vi "Remove Connection.vi"(8 "error in (no error)":errorcluster, 11 "Terminal in":refnum<class "Terminal.lvclass">) -> (0 "error out":errorcluster, 2 "Connection":refnum<class "Connection.lvclass">, 3 "Terminal out":refnum<class "Terminal.lvclass">)   [LabVIEW 2020, in "Terminal.lvlib" / "Terminal.lvclass"]
uses:
  Terminal.lvclass
  Terminal.lvclass/Terminal.ctl
  Connection State Callback.vi
  Data Sniffer Callback.vi
  <vilib>/IlluminatedG/lv-stream/Endpoint/Endpoint.lvclass
  <vilib>/IlluminatedG/lv-stream/Connection/Connection.lvclass
  C:/Program Files (x86)/National Instruments/LabVIEW 2020/vi.lib/IlluminatedG/lv-stream/Endpoint/Endpoint.lvclass
  C:/Program Files (x86)/National Instruments/LabVIEW 2020/vi.lib/IlluminatedG/lv-stream/Connection/Connection.lvclass
  C:/Program Files (x86)/National Instruments/LabVIEW 2020/vi.lib/IlluminatedG/IG OOPanel/OOPanel/Panel/Panel.lvclass
  C:/dev/illuminated-g/lv-stream-terminal/Terminal/Terminal/Terminal.lvclass
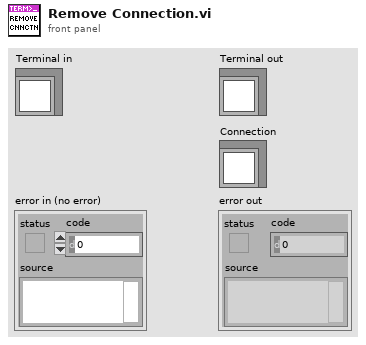
[diagram p1: front panel]
types:
  T1 = typedef "Terminal.lvlib/Terminal.lvclass/Ref Data.ctl" = cluster{"Connection":refnum<class "Connection.lvclass">, "Read Loop Running":bool, "Parse State":T2, "Terminal Options":T8, "Font Metrics":T11, "Scroll":i32, "Close Read Loop":bool, "Buffer":T7, "Pause Read Loop":bool, "User Input Enabled":bool, "Cursor Enabled":bool, "Cursor Blink":bool}
  T2 = typedef "Terminal.lvlib/Terminal.lvclass/Parse State.ctl" = cluster{"Buffer State":T3, "Cursor":T4, "Attributes":T6, "Active Buffer":T7}
  T3 = typedef "Terminal.lvlib/Terminal.lvclass/Buffer State.ctl" = cluster{"Sequence":string, "ESC":bool, "Alt Buf":bool}
  T4 = typedef "Terminal.lvlib/Terminal.lvclass/Cursor.ctl" = cluster{"Cur":T5, "Saved":T5}
  T5 = typedef "Terminal.lvlib/Terminal.lvclass/Position.ctl" = cluster{"Row":i32, "Col":i32}
  T6 = typedef "Terminal.lvlib/Text Attributes.ctl" = cluster{"FG":u32, "BG":u32, "Bold":bool, "Italic":bool, "Underline":bool, "Strike":bool, "Inverse":bool}
  T7 = typedef "Terminal.lvlib/Buffer.ctl" = enum16{"Primary", "Alternate"}
  T8 = typedef "Terminal.lvlib/Terminal Options.ctl" = cluster{"Implied CR with LF":bool, "Local Echo":bool, "Tab Width":i32, "Color Scheme":T9, "Default FG":T10, "Default BG":T10, "History Length":i32, "Font Face":string, "Font Size":i16, "Rows":i32, "Cols":i32}
  T9 = typedef "Terminal.lvlib/Color Scheme.ctl" = cluster{"Black":u32, "Red":u32, "Green":u32, "Yellow":u32, "Blue":u32, "Magenta":u32, "Cyan":u32, "White":u32, "Bright Black":u32, "Bright Red":u32, "Bright Green":u32, "Bright Yellow":u32, "Bright Blue":u32, "Bright Magenta":u32, "Bright Cyan":u32, "Bright White":u32}
  T10 = typedef "Terminal.lvlib/Color.ctl" = i8
  T11 = typedef "Terminal.lvlib/Terminal.lvclass/Font Metrics.ctl" = cluster{"Width":i16, "Height":i16}
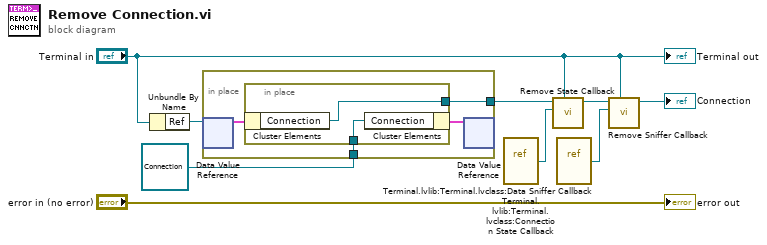
[diagram p0: block diagram]
diagram:
  n1 = Unbundle By Name("Terminal in") -> ("Ref"=w9:refnum<data-value>)
  n2 = in-place {
    in-place-border: [w11] -> w8
    in-place-border: refnum<class "Connection.lvclass"> refnum ("Connection") -> [w10]
    n3 = in-place-dvr #1(w9) -> (w13:T1)  [unwired: 1 out]
    n4 = in-place {
      in-place-border: [w15] -> w11
      in-place-border: w10 -> [w14]
      n5 = in-place-cluster #2(w13) -> ("Connection"=w15:refnum<class "Connection.lvclass">)
      n6 = in-place-cluster #2("Connection"=w14) -> (w12:T1)
    }
    n7 = in-place-dvr #1(w12) -> ()  [unwired: 2 out]
  }
  n8 = vi-ref "Terminal.lvlib:Terminal.lvclass:Connection State Callback.vi"() -> (w7:refnum<vi>)
  n9 = call <vilib>:"Remove State Callback.vi"("Owner (None)"="Terminal in", "Callback"=w7, "Endpoint in"=w8) -> ("Endpoint out"=w6:refnum<class "Connection.lvclass">)  [unwired: 6 in, 2 out]
  n10 = vi-ref "Terminal.lvlib:Terminal.lvclass:Data Sniffer Callback.vi"() -> (w5:refnum<vi>)
  n11 = call <vilib>:"Remove Sniffer Callback.vi"("Owner"="Terminal in", "Callback"=w5, "Endpoint in"=w6) -> ("Endpoint out"=→"Connection":refnum<class "Connection.lvclass">)  [unwired: 7 in, 1 out]
  "error out" <- "error in (no error)"
  "Terminal out" <- "Terminal in"
